vi "Excel Example.vi"() -> ()   [LabVIEW 2017]
uses:
  LabVIEW NPOI/Document/Document.lvclass
  LabVIEW NPOI/MS-Excel/MS-Excel.lvclass
  LabVIEW NPOI/Document/Append Table (string).vi
  LabVIEW NPOI/Document/Append Table (double).vi
  Styles/Underline--ring.ctl
  Styles/Styles.lvlib
  Styles/Alignment--ring.ctl
  Styles/Font--cluster.ctl
  Styles/Style--cluster.ctl
  LabVIEW NPOI/Document/Read Table As String.vi
  D:/Benjamin/Documents/Perso/Code/WC/LabVIEW_NPOI/src/LabVIEW NPOI/Document/Document.lvclass
panel:
  in  "setActiveSheetBttn":bool
  out "Table Control":string[][](table)
  in  "readTableBttn":bool
  in  "Style":u16(ring) items=["Default", "Heading 1", "Heading 2", "Heading 3", "Title"]
  out "Current Sheet:Next Empty Cell":cluster{"Row":i32, "Column":i32}
  in  "#Columns":i32=100
  in  "#Rows":i32=2
  in  "tableType":enum32{"Strings", "Doubles"}(radio)
  in  "addTableBttn":bool
  in  "Set as active (T)":bool
  in  "addWorksheetBttn":bool
  out "Current Sheet:Name":string
  out "Workbook:Sheet List":string[](array[string])
  out "FilePath":path
  in  "openWorkbookBttn":bool
  in  "baseWorkbookPath":path caption="Folder Path"
  in  "saveAsWorkbookBttn":bool
  in  "saveWorkbookBttn":bool
  in  "removeSheetBttn":bool
  in  "workbookName":string="Book1.xlsx" caption="Name"
  in  "newWorksheetName":string caption="Sheet Name"
  in  "createWorkbookBttn":bool
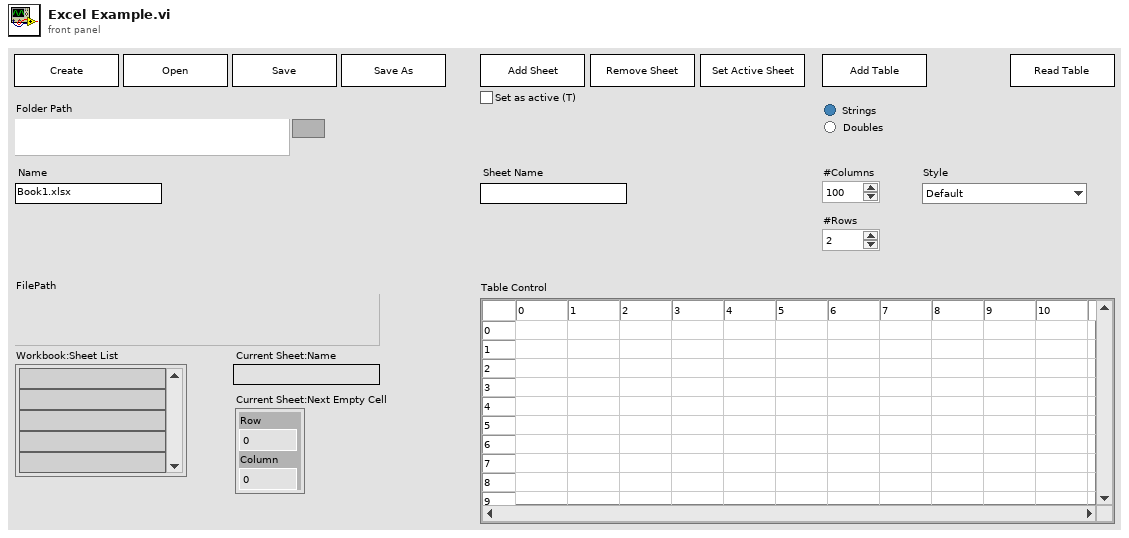
[diagram p1: front panel]
types:
  T1 = cluster{"workbookObject":refnum<class "MS-Excel.lvclass">, "workbookPath":path, "workbookName":string, "worksheetName":string, "styleName":string, "ctlRefs":refnum<vi>[]}
  T2 = typedef "Styles.lvlib/Style--cluster.ctl" = cluster{"Name":string, "Font":T3}
  T3 = typedef "Styles.lvlib/Font--cluster.ctl" = cluster{"Name":string, "Size":i32, "Bold":bool, "Italic":bool, "Underline":T4, "Strike":bool, "Color":u32, "Alignment":T5}
  T4 = typedef "Styles.lvlib/Underline--ring.ctl" = i32
  T5 = typedef "Styles.lvlib/Alignment--ring.ctl" = i32
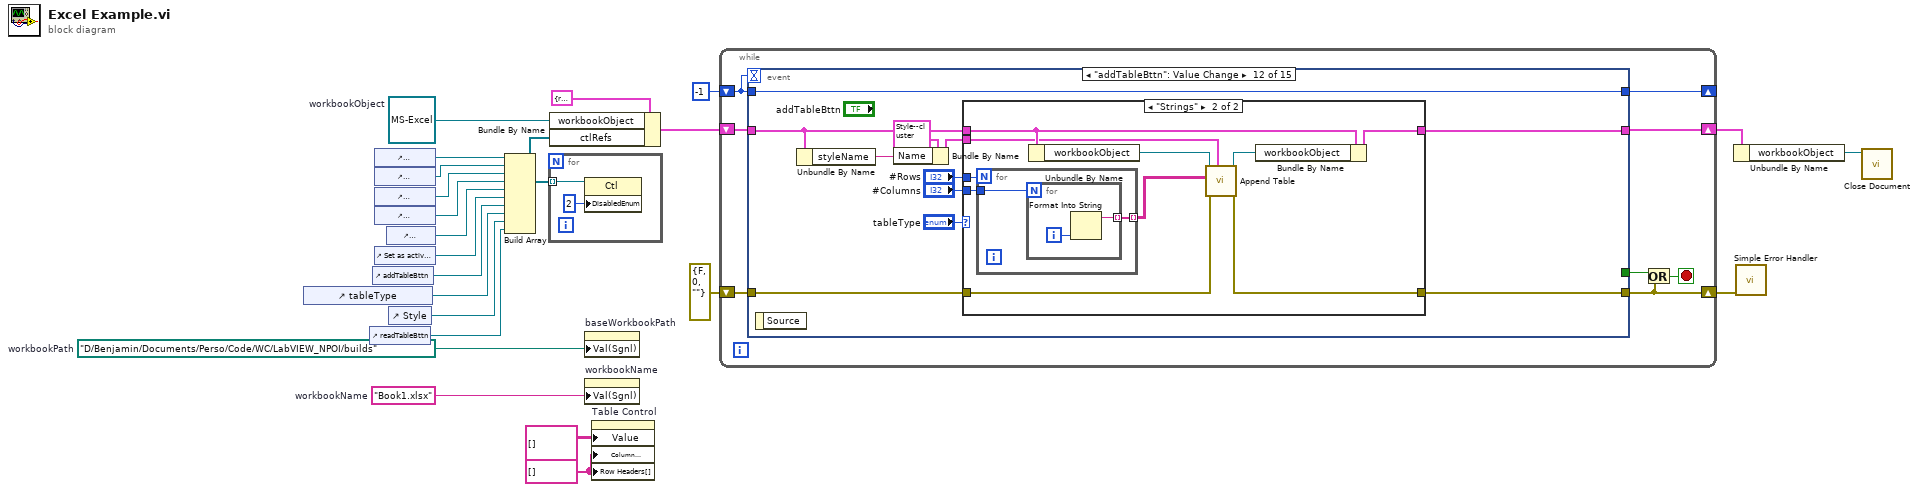
[diagram p0: block diagram]
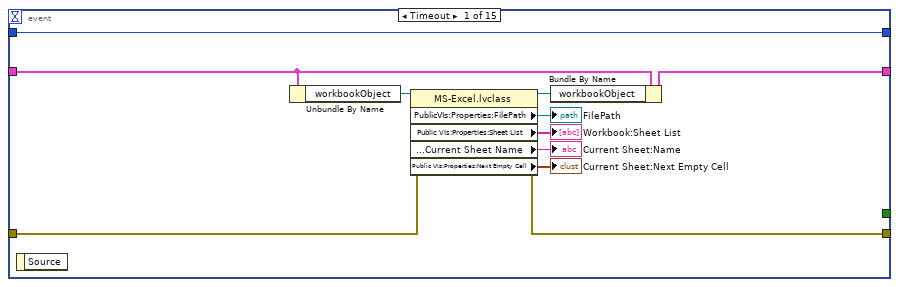
[diagram p2: hidden frame]
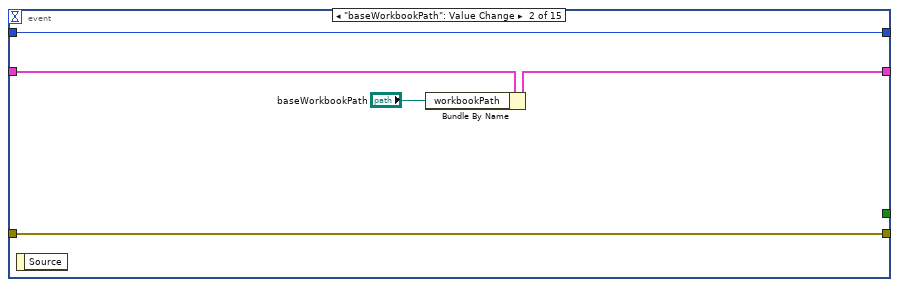
[diagram p3: hidden frame]
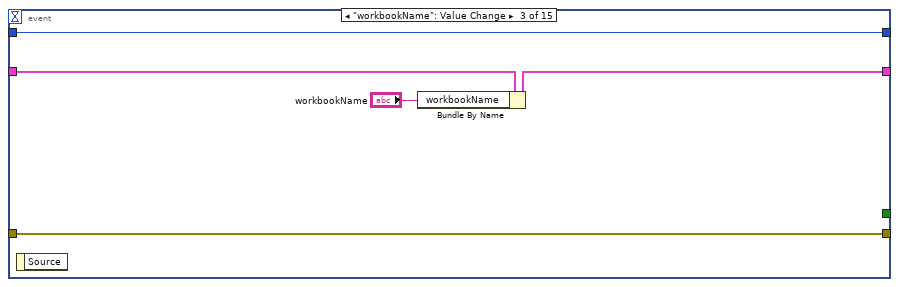
[diagram p4: hidden frame]
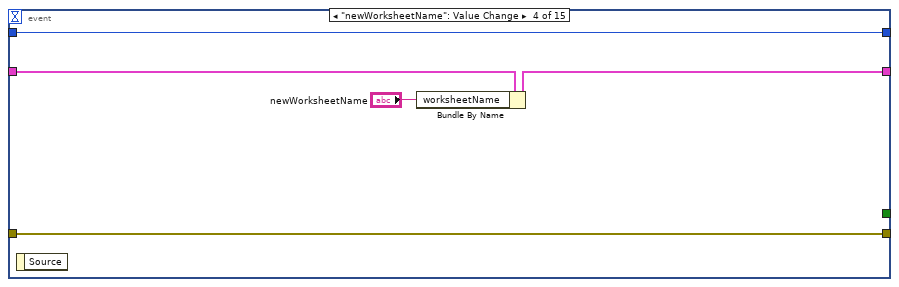
[diagram p5: hidden frame]
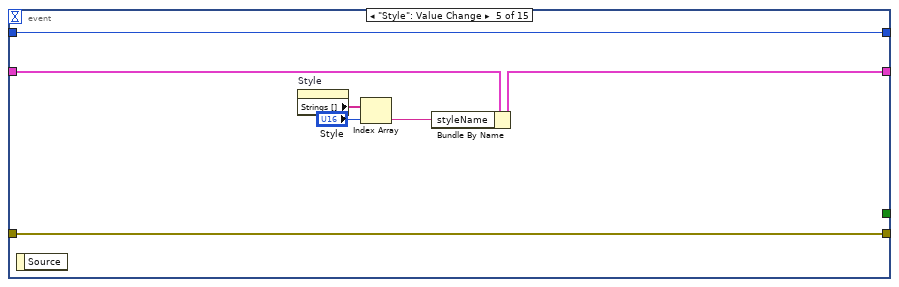
[diagram p6: hidden frame]
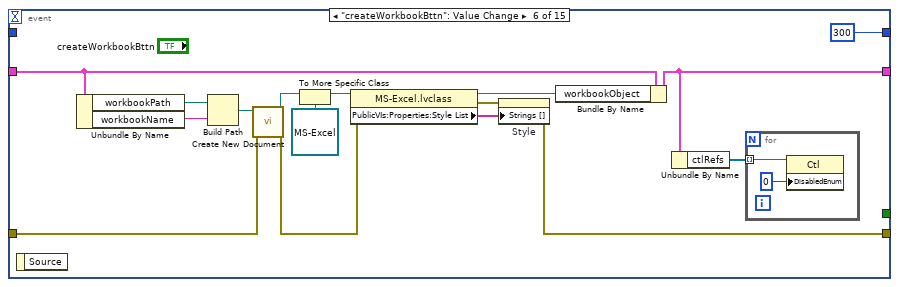
[diagram p7: hidden frame]
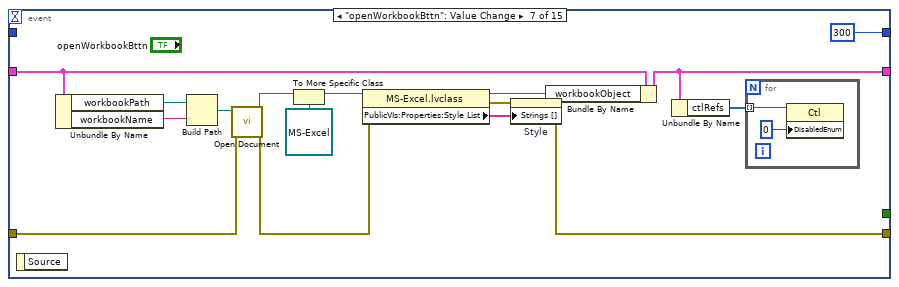
[diagram p8: hidden frame]
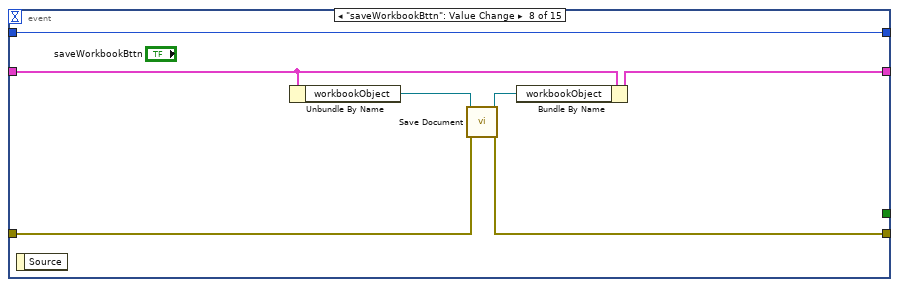
[diagram p9: hidden frame]
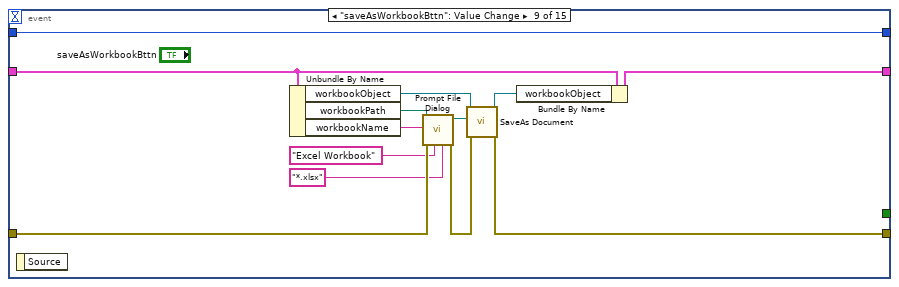
[diagram p10: hidden frame]
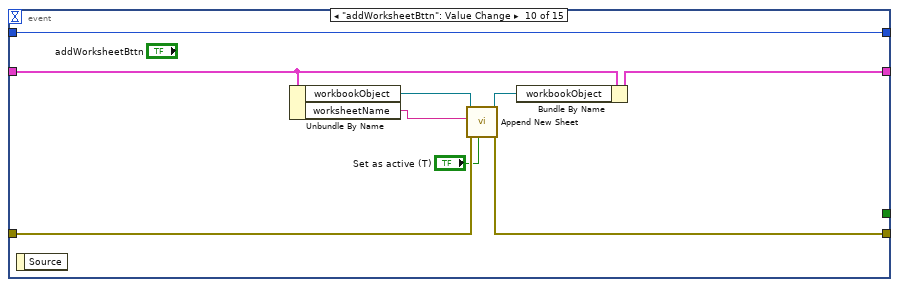
[diagram p11: hidden frame]
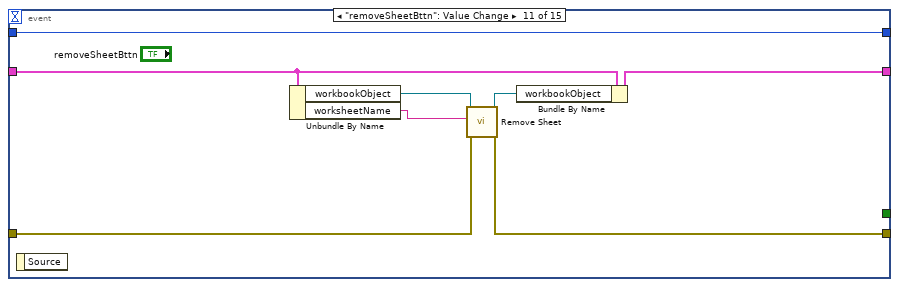
[diagram p12: hidden frame]
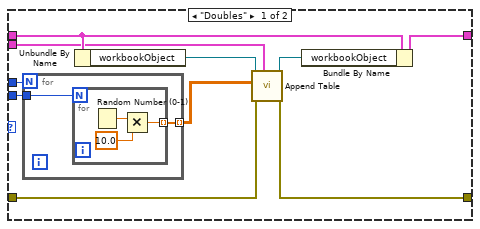
[diagram p13: hidden frame]
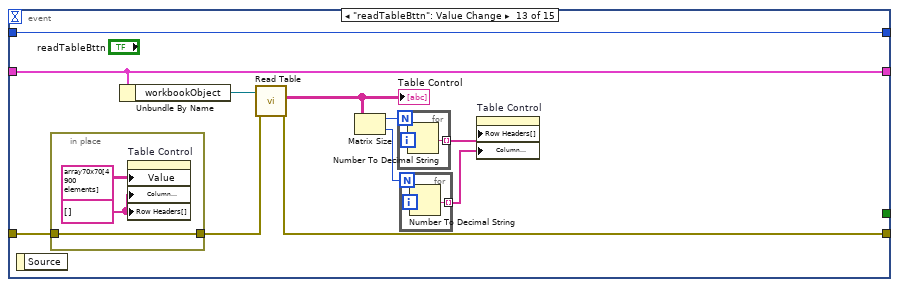
[diagram p14: hidden frame]
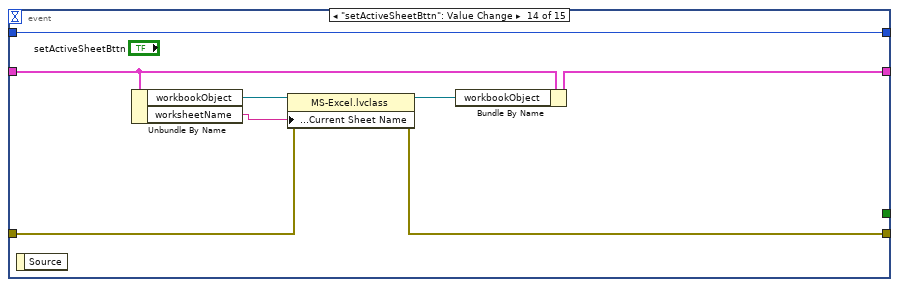
[diagram p15: hidden frame]
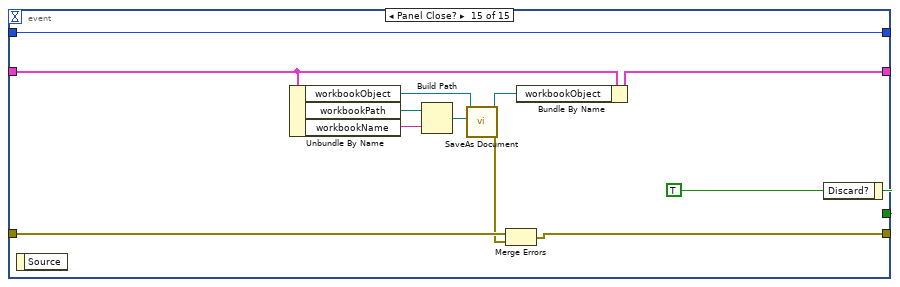
[diagram p16: hidden frame]
diagram:
  w1 = string[] [] ("Row Header Strings[]")
  w7 = "Book1.xlsx"  # workbookName
  w8 = path "D:/Benjamin/Documents/Perso/Code/WC/LabVIEW_NPOI/builds"  # workbookPath
  w16 = refnum<class "MS-Excel.lvclass"> refnum  # workbookObject
  n1 = control-ref of="tableType"() -> (w5:refnum<vi>)
  n2 = control-ref of="readTableBttn"() -> (w3:refnum<vi>)
  n3 = control-ref of="addTableBttn"() -> (w6:refnum<vi>)
  n4 = control-ref of="saveWorkbookBttn"() -> (w15:refnum<vi>)
  n5 = control-ref of="saveAsWorkbookBttn"() -> (w14:refnum<vi>)
  n6 = control-ref of="addWorksheetBttn"() -> (w13:refnum<vi>)
  n7 = control-ref of="removeSheetBttn"() -> (w12:refnum<vi>)
  n8 = control-ref of="Set as active (T)"() -> (w10:refnum<vi>)
  n9 = control-ref of="newWorksheetName"() -> (w11:refnum<vi>)
  n10 = control-ref of="Style"() -> (w4:refnum<vi>)
  n11 = Build Array(w15, w14, w13, w12, w11, w10, w6, w5, w4, w3) -> (w9:refnum<vi>[])
  n12 = for {
    tunnel: w9 -> [w25] mode=indexing
    n13 = property class="Ctl"(reference=w25, "DisabledEnum"=u8 2) -> ()  [unwired: 1 in, 2 out]
  }
  n14 = Bundle By Name(cluster=T1 {"workbookObject"=refnum, "workbookPath"=path "", "workbookName"="", "worksheetName"="", "styleName"="Default", "ctlRefs"=[]}, "workbookObject"=w16, "ctlRefs"=w9) -> (w23:T1)
  n15 = property on="baseWorkbookPath" class="Path"("Val(Sgnl)"=w8) -> ()  [unwired: 2 in, 2 out]
  n16 = property on="workbookName" class="Str"("Val(Sgnl)"=w7) -> ()  [unwired: 2 in, 2 out]
  n17 = property on="Table Control" class="Tbl (strict)"("Value"=string[][] [] ("Table Control"), "Column Headers[]"=w1, "Row Headers[]"=w1) -> ()  [unwired: 2 in, 2 out]
  n18 = while {
    shift-right: [w32] -> w19
    shift-left: w23 -> [w33]
    shift-right: [w30] -> w22
    shift-left: errorcluster {"status"=FALSE, "code"=0, "source"=""} ("error IO") -> [w31]
    shift-right: [w26] -> _
    shift-left: -1 -> [w27]
    stop <- w28 stop-if-true
    n19 = event shown="[11] \"addTableBttn\": Value Change" {
      selector: _ -> [_ _ _ _ _ _ _ _ _ _ _ _ _ _ _]
      dyn-events: _ -> [_ _ _ _ _ _ _ _ _ _ _ _ _ _ _]
      timeout: w27 -> [_ _ _ _ _ _ _ _ _ _ _ _ _ _ _]
      tunnel: [_ _ _ _ _ _ _ _ _ _ _ _ _ _ w210] -> w29
      tunnel: w33 -> [w44 w49 w54 w59 w66 w82 w100 w109 w122 w131 w139 w143 w189 w204 w217]
      tunnel: [w35 w48 w53 w57 w64 w76 w95 w107 w120 w129 w137 w150 w189 w199 w212] -> w32
      tunnel: [w40 w46 w51 w58 w65 w70 w89 w105 w118 w127 w135 w149 w187 w200 w208] -> w30
      tunnel: w31 -> [w41 w46 w51 w58 w65 w78 w97 w104 w116 w126 w134 w148 w181 w201 w209]
      tunnel: w27 -> [w36 w45 w50 w55 w63 _ _ w103 w110 w124 w132 w147 w190 w205 w206]
      tunnel: [w36 w45 w50 w55 w63 300 300 w103 w110 w124 w132 w147 w190 w205 w206] -> w26
      event Timeout {
        n20 = event-data() -> ()  [unwired: 1 in, 1 out]
        n21 = Unbundle By Name(w44) -> ("workbookObject"=w43:refnum<class "MS-Excel.lvclass">)
        n22 = property class="MS-Excel.lvclass"(reference=w43, error in=w41) -> (reference out=w42:refnum<class "MS-Excel.lvclass">, error out=w40:errorcluster, "PublicVIs:Properties:FilePath"=→"FilePath":path, "Public VIs:Properties:Sheet List"=→"Workbook:Sheet List":string[], "Public VIs:Properties:Current Sheet Name"=→"Current Sheet:Name":string, "Public VIs:Properties:Next Empty Cell"=→"Current Sheet:Next Empty Cell":cluster{"Row":i32, "Column":i32})
        n23 = Bundle By Name(cluster=w44, "workbookObject"=w42) -> (w35:T1)
      }
      event "baseWorkbookPath": Value Change {
        n24 = event-data() -> ()  [unwired: 1 in, 1 out]
        n25 = Bundle By Name(cluster=w49, "workbookPath"="baseWorkbookPath") -> (w48:T1)
      }
      event "workbookName": Value Change {
        n26 = event-data() -> ()  [unwired: 1 in, 1 out]
        n27 = Bundle By Name(cluster=w54, "workbookName"="workbookName") -> (w53:T1)
      }
      event "newWorksheetName": Value Change {
        n28 = event-data() -> ()  [unwired: 1 in, 1 out]
        n29 = Bundle By Name(cluster=w59, "worksheetName"="newWorksheetName") -> (w57:T1)
      }
      event "Style": Value Change {
        n30 = event-data() -> ()  [unwired: 1 in, 1 out]
        n31 = property on="Style" class="Ring (strict)"() -> ("Strings []"=w62:string[])  [unwired: 2 in, 2 out]
        n32 = Index Array(array=w62, index="Style") -> (element=w61:string)
        n33 = Bundle By Name(cluster=w66, "styleName"=w61) -> (w64:T1)
      }
      event "createWorkbookBttn": Value Change {
        n34 = event-data() -> ()  [unwired: 1 in, 1 out]
        n35 = Unbundle By Name(w82) -> ("workbookPath"=w81:path, "workbookName"=w80:string)
        n36 = Build Path(base path=w81, name or relative path=w80) -> (appended path=w69:path)
        n37 = call "Create New Document.vi"("error in (no error)"=w78, "File Path"=w69) -> ("error out"=w73:errorcluster, "Document out"=w79:refnum<class "Document.lvclass">)  [unwired: 8 in]
        n38 = To More Specific Class(target class=refnum<class "MS-Excel.lvclass"> refnum ("workbookObject"), reference=w79) -> (specific class reference=w68:refnum<class "MS-Excel.lvclass">)  [unwired: 1 in, 1 out]
        n39 = property class="MS-Excel.lvclass"(reference=w68, error in=w73) -> (reference out=w74:refnum<class "MS-Excel.lvclass">, error out=w71:errorcluster, "PublicVIs:Properties:Style List"=w72:string[])
        n40 = property on="Style" class="Ring (strict)"(error in=w71, "Strings []"=w72) -> (error out=w70:errorcluster)  [unwired: 1 in, 1 out]
        n41 = Bundle By Name(cluster=w82, "workbookObject"=w74) -> (w76:T1)
        n42 = Unbundle By Name(w76) -> ("ctlRefs"=w75:refnum<vi>[])
        n43 = for {
          tunnel: w75 -> [w84] mode=indexing
          n44 = property class="Ctl"(reference=w84, "DisabledEnum"=u8 0) -> ()  [unwired: 1 in, 2 out]
        }
      }
      event "openWorkbookBttn": Value Change {
        n45 = event-data() -> ()  [unwired: 1 in, 1 out]
        n46 = Unbundle By Name(w100) -> ("workbookPath"=w99:path, "workbookName"=w98:string)
        n47 = Build Path(base path=w99, name or relative path=w98) -> (appended path=w88:path)
        n48 = call "Open Document.vi"("error in (no error)"=w97, "File Path"=w88) -> ("error out"=w91:errorcluster, "Document out"=w86:refnum<class "Document.lvclass">)  [unwired: 8 in]
        n49 = To More Specific Class(target class=refnum<class "MS-Excel.lvclass"> refnum ("workbookObject"), reference=w86) -> (specific class reference=w85:refnum<class "MS-Excel.lvclass">)  [unwired: 1 in, 1 out]
        n50 = property class="MS-Excel.lvclass"(reference=w85, error in=w91) -> (reference out=w92:refnum<class "MS-Excel.lvclass">, error out=w90:errorcluster, "PublicVIs:Properties:Style List"=w93:string[])
        n51 = property on="Style" class="Ring (strict)"(error in=w90, "Strings []"=w93) -> (error out=w89:errorcluster)  [unwired: 1 in, 1 out]
        n52 = Bundle By Name(cluster=w100, "workbookObject"=w92) -> (w95:T1)
        n53 = Unbundle By Name(w95) -> ("ctlRefs"=w94:refnum<vi>[])
        n54 = for {
          tunnel: w94 -> [w102] mode=indexing
          n55 = property class="Ctl"(reference=w102, "DisabledEnum"=u8 0) -> ()  [unwired: 1 in, 2 out]
        }
      }
      event "saveWorkbookBttn": Value Change {
        n56 = event-data() -> ()  [unwired: 1 in, 1 out]
        n57 = Unbundle By Name(w109) -> ("workbookObject"=w108:refnum<class "MS-Excel.lvclass">)
        n58 = call "Save Document.vi"("error in (no error)"=w104, "Document in"=w108) -> ("error out"=w105:errorcluster, "Document out"=w106:refnum<class "MS-Excel.lvclass">)  [unwired: 8 in]
        n59 = Bundle By Name(cluster=w109, "workbookObject"=w106) -> (w107:T1)
      }
      event "saveAsWorkbookBttn": Value Change {
        n60 = event-data() -> ()  [unwired: 1 in, 1 out]
        n61 = Unbundle By Name(w122) -> ("workbookObject"=w121:refnum<class "MS-Excel.lvclass">, "workbookPath"=w112:path, "workbookName"=w111:string)
        n62 = call "Prompt File Dialog.vi"("pattern (all files)"="*.xlsx", "pattern label"="Excel Workbook", "error in"=w116, "default name"=w111, "File Path"=w112) -> ("error out"=w115:errorcluster, "selected path"=w117:path)  [unwired: 5 in]
        n63 = call "SaveAs Document.vi"("error in (no error)"=w115, "File Path"=w117, "Document in"=w121) -> ("error out"=w118:errorcluster, "Document out"=w119:refnum<class "MS-Excel.lvclass">)  [unwired: 7 in]
        n64 = Bundle By Name(cluster=w122, "workbookObject"=w119) -> (w120:T1)
      }
      event "addWorksheetBttn": Value Change {
        n65 = event-data() -> ()  [unwired: 1 in, 1 out]
        n66 = Unbundle By Name(w131) -> ("workbookObject"=w130:refnum<class "MS-Excel.lvclass">, "worksheetName"=w125:string)
        n67 = call "Append New Sheet.vi"("Set as active (T)"="Set as active (T)", "error in (no error)"=w126, "Sheet Name"=w125, "MS-Excel in"=w130) -> ("error out"=w127:errorcluster, "MS-Excel out"=w128:refnum<class "MS-Excel.lvclass">)  [unwired: 4 in, 2 out]
        n68 = Bundle By Name(cluster=w131, "workbookObject"=w128) -> (w129:T1)
      }
      event "removeSheetBttn": Value Change {
        n69 = event-data() -> ()  [unwired: 1 in, 1 out]
        n70 = Unbundle By Name(w139) -> ("workbookObject"=w138:refnum<class "MS-Excel.lvclass">, "worksheetName"=w133:string)
        n71 = call "Remove Sheet.vi"("error in (no error)"=w134, "Sheet Name"=w133, "MS-Excel in"=w138) -> ("error out"=w135:errorcluster, "MS-Excel out"=w136:refnum<class "MS-Excel.lvclass">)  [unwired: 7 in]
        n72 = Bundle By Name(cluster=w139, "workbookObject"=w136) -> (w137:T1)
      }
      event "addTableBttn": Value Change {
        n73 = event-data() -> ()  [unwired: 1 in, 1 out]
        n74 = Unbundle By Name(w143) -> ("styleName"=w140:string)
        n75 = Bundle By Name(cluster=T2 {"Name"="Default", "Font"={"Name"="Calibri", "Size"=12, "Bold"=FALSE, "Italic"=FALSE, "Underline"=18, "Strike"=FALSE, "Color"=0, "Alignment"=1}} ("Style"), "Name"=w140) -> (w141:T2)
        n76 = case shown="\"Strings\"" "tableType" {
          tunnel: w143 -> [w160 w175]
          tunnel: [w158 w173] -> w150
          tunnel: [w156 w171] -> w149
          tunnel: w148 -> [w155 w170]
          tunnel: "#Columns" -> [w152 w168]
          tunnel: "#Rows" -> [w153 w167]
          tunnel: w141 -> [w151 w166]
          frame "Doubles" {
            n77 = for {
              N: w153 -> [_]
              tunnel: [w162] -> w154 mode=indexing
              tunnel: w152 -> [w161]
              n78 = for {
                N: w161 -> [_]
                tunnel: [w164] -> w162 mode=indexing
                n79 = Random Number (0-1)() -> (number: 0 to 1=w165:dbl)
                n80 = Multiply(x=w165, y=10.0) -> (x*y=w164:dbl)
              }
            }
            n81 = Unbundle By Name(w160) -> ("workbookObject"=w159:refnum<class "MS-Excel.lvclass">)
            n82 = call-poly "Append Table.vi"("Style"=w151, "error in (no error)"=w155, "Table"=w154, "Document in"=w159) -> ("error out"=w156:errorcluster, "Document out"=w157:refnum<class "MS-Excel.lvclass">)  [unwired: 6 in]
            n83 = Bundle By Name(cluster=w160, "workbookObject"=w157) -> (w158:T1)
          }
          frame "Strings" {
            n84 = for {
              N: w167 -> [_]
              tunnel: [w177] -> w169 mode=indexing
              tunnel: w168 -> [w176]
              n85 = for {
                N: w176 -> [_]
                tunnel: [w178] -> w177 mode=indexing
                i -> [w179]
                n86 = Format Into String(w179) -> (resulting string=w178:string)  [unwired: 3 in, 1 out]
              }
            }
            n87 = Unbundle By Name(w175) -> ("workbookObject"=w174:refnum<class "MS-Excel.lvclass">)
            n88 = call-poly "Append Table.vi"("Style"=w166, "error in (no error)"=w170, "Table"=w169, "Document in"=w174) -> ("error out"=w171:errorcluster, "Document out"=w172:refnum<class "MS-Excel.lvclass">)  [unwired: 6 in]
            n89 = Bundle By Name(cluster=w175, "workbookObject"=w172) -> (w173:T1)
          }
        }
      }
      event "readTableBttn": Value Change {
        n90 = event-data() -> ()  [unwired: 1 in, 1 out]
        n91 = in-place {
          in-place-border: w181 -> [w191]
          in-place-border: [w191] -> w180
          w193 = string[] [] ("Row Header Strings[]")
          n92 = property on="Table Control" class="Tbl (strict)"("Value"=string[][] array70x70[4900 elements] ("Table Control"), "Column Headers[]"=w193, "Row Headers[]"=w193) -> ()  [unwired: 2 in, 2 out]
        }
        n93 = Unbundle By Name(w189) -> ("workbookObject"=w188:refnum<class "MS-Excel.lvclass">)
        n94 = call-poly "Read Table.vi"("error in (no error)"=w180, "Document in"=w188) -> ("error out"=w187:errorcluster, "Table As String"=w186:string[][])  [unwired: 7 in, 1 out]
        "Table Control" <- w186
        n95 = Matrix Size(0:w186) -> (1:w185:i32, 2:w183:i32)
        n96 = for {
          N: w185 -> [_]
          tunnel: [w196] -> w184 mode=indexing
          i -> [w197]
          n97 = Number To Decimal String(number=w197) -> (decimal integer string=w196:string)  [unwired: 1 in]
        }
        n98 = for {
          N: w183 -> [_]
          tunnel: [w194] -> w182 mode=indexing
          i -> [w195]
          n99 = Number To Decimal String(number=w195) -> (decimal integer string=w194:string)  [unwired: 1 in]
        }
        n100 = property on="Table Control" class="Tbl (strict)"("Row Headers[]"=w184, "Column Headers[]"=w182) -> ()  [unwired: 2 in, 2 out]
      }
      event "setActiveSheetBttn": Value Change {
        n101 = event-data() -> ()  [unwired: 1 in, 1 out]
        n102 = Unbundle By Name(w204) -> ("workbookObject"=w203:refnum<class "MS-Excel.lvclass">, "worksheetName"=w202:string)
        n103 = property class="MS-Excel.lvclass"(reference=w203, error in=w201, "Public VIs:Properties:Current Sheet Name"=w202) -> (reference out=w198:refnum<class "MS-Excel.lvclass">, error out=w200:errorcluster)
        n104 = Bundle By Name(cluster=w204, "workbookObject"=w198) -> (w199:T1)
      }
      event Panel Close? {
        w210 = TRUE ("Discard?")
        n105 = event-data() -> ()  [unwired: 1 in, 1 out]
        n106 = Unbundle By Name(w217) -> ("workbookObject"=w214:refnum<class "MS-Excel.lvclass">, "workbookPath"=w216:path, "workbookName"=w215:string)
        n107 = Build Path(base path=w216, name or relative path=w215) -> (appended path=w213:path)
        n108 = call "SaveAs Document.vi"("File Path"=w213, "Document in"=w214) -> ("error out"=w207:errorcluster, "Document out"=w211:refnum<class "MS-Excel.lvclass">)  [unwired: 8 in]
        n109 = Merge Errors(w209, w207) -> (w208:errorcluster)
        n110 = Bundle By Name(cluster=w217, "workbookObject"=w211) -> (w212:T1)
        n111 = event-data("Discard?"=w210) -> ()  [unwired: 1 in, 1 out]
      }
    }
    n112 = Or(x=w29, y=w30) -> (x .or. y?=w28:bool)
  }
  n113 = Unbundle By Name(w19) -> ("workbookObject"=w18:refnum<class "MS-Excel.lvclass">)
  n114 = call <vilib>:"Simple Error Handler.vi"("error in (no error)"=w22) -> ()  [unwired: 4 in, 5 out]
  n115 = call "Close Document.vi"("Document in"=w18) -> ()  [unwired: 10 in, 1 out]
